vi "Salidas_digitales.vi"() -> ()   [LabVIEW 2023]
uses:
  <vilib>/Instr/_visa.llb/VISA Configure Serial Port (Instr).vi
panel:
  out "String":string
  in  "stop":bool
  in  "VISA resource name":refnum<visa-resource-name>
  in  "S4":bool
  in  "S3":bool
  in  "S2":bool
  in  "S1":bool
  # "Salidas Digitales"
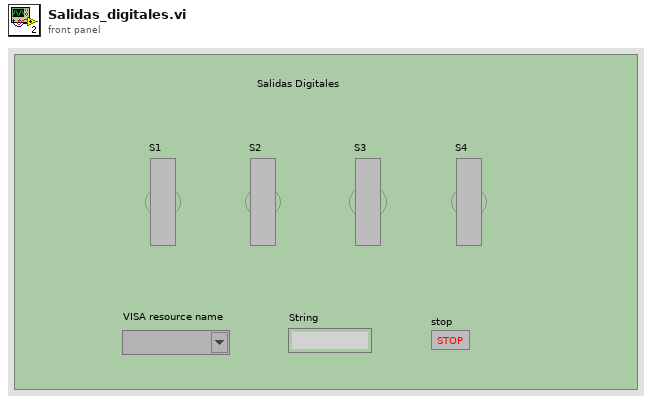
[diagram p1: front panel]
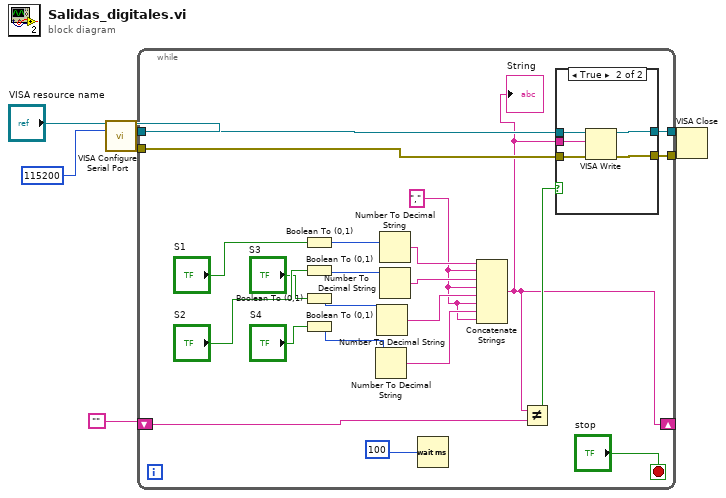
[diagram p0: block diagram]
diagram:
  n1 = call-poly "VISA Configure Serial Port"("VISA resource name"="VISA resource name", "baud rate (9600)"=u32 115200) -> ("VISA resource name out"=w6:refnum<visa-resource-name>, "error out"=w4:errorcluster)  [unwired: 12 in]
  n2 = while {
    tunnel: w6 -> [w29]
    tunnel: [w28] -> w5
    tunnel: w4 -> [w27]
    tunnel: [w26] -> w3
    shift-right: [w11] -> _
    shift-left: "" -> [w13]
    stop <- "stop" stop-if-true
    w8 = ","
    n3 = Boolean To (0,1)(Boolean="S1") -> (0, 1=w21:i16)
    n4 = Boolean To (0,1)(Boolean="S2") -> (0, 1=w20:i16)
    n5 = Boolean To (0,1)(Boolean="S3") -> (0, 1=w19:i16)
    n6 = Boolean To (0,1)(Boolean="S4") -> (0, 1=w18:i16)
    n7 = Number To Decimal String(number=w18) -> (decimal integer string=w14:string)  [unwired: 1 in]
    n8 = Number To Decimal String(number=w19) -> (decimal integer string=w15:string)  [unwired: 1 in]
    n9 = Number To Decimal String(number=w21) -> (decimal integer string=w17:string)  [unwired: 1 in]
    n10 = Number To Decimal String(number=w20) -> (decimal integer string=w16:string)  [unwired: 1 in]
    n11 = Wait (ms)(milliseconds to wait=u32 100 ("millisecond timer value")) -> ()  [unwired: 1 out]
    n12 = Concatenate Strings(w17, w8, w16, w8, w15, w8, w14, w8) -> (w11:string)
    "String" <- w11
    n13 = Not Equal?(x=w11, y=w13) -> (x != y?=w12:bool)
    n14 = case shown="True" w12 {
      tunnel: w29 -> [w31 w36]
      tunnel: [w31 w35] -> w28
      tunnel: w27 -> [w30 w34]
      tunnel: [w30 w33] -> w26
      tunnel: w11 -> [_ w32]
      frame False {
      }
      frame True {
        n15 = VISA Write(VISA resource name=w36, write buffer=w32, error in (no error)=w34) -> (VISA resource name out=w35:refnum<visa-resource-name>, error out=w33:errorcluster)  [unwired: 1 out]
      }
    }
  }
  n16 = VISA Close(VISA resource name=w5, error in (no error)=w3) -> ()  [unwired: 1 out]
